vi "Get Volts.vi"(8 "error in (no error)":errorcluster, 11 "Multimetro in":refnum<class "Multimetro.lvclass">) -> (0 "error out":errorcluster, 2 "Volts":dbl, 3 "Multimetro out":refnum<class "Multimetro.lvclass">)   [LabVIEW 2020, in "Multimetro.lvclass"]
uses:
  Multimetro.lvclass
  Multimetro.lvclass/Multimetro.ctl
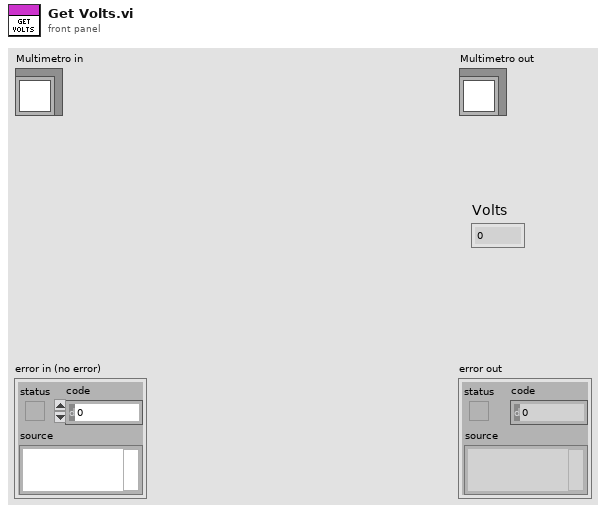
[diagram p1: front panel]
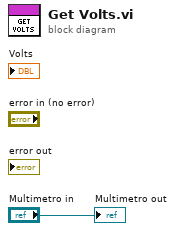
[diagram p0: block diagram]
diagram:
  "Multimetro out" <- "Multimetro in"
